vi "ActuatorMotor.vi"(4 "Actuator Name":string, 5 "Command":T1(ring)=enum."GetAbsolutePosition", 6 "error in (no error)":errorcluster, 8 "Y":dbl, 9 "X":dbl) -> (0 "error out":errorcluster, 2 "Y out":dbl, 3 "X out":dbl)   [LabVIEW 2009]
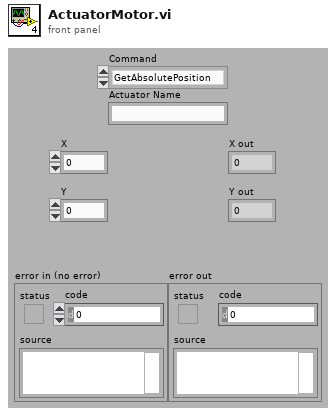
[diagram p1: front panel]
types:
  T1 = enum16{"Acquire", "GetAbsolutePosition", "AbsoluteMove", "Release"}
  T2 = typedef "MotorStatus.ctl" = cluster{"Managed?":bool, "Position":i32, "Name":string, "Status":enum16{"OFF", "IDLE", "MOVING", "HOMING"}}
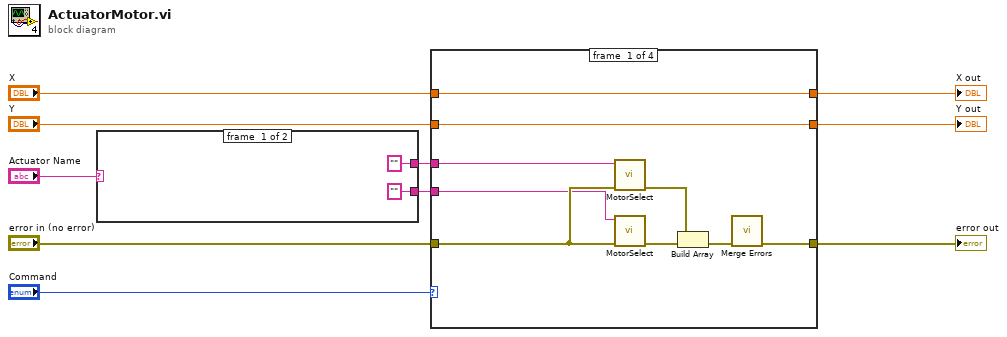
[diagram p0: block diagram]
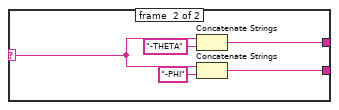
[diagram p2: hidden frame]
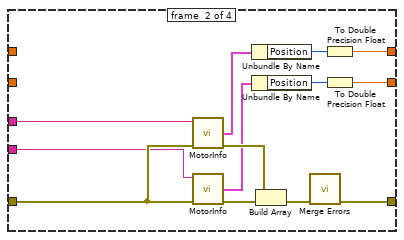
[diagram p3: hidden frame]
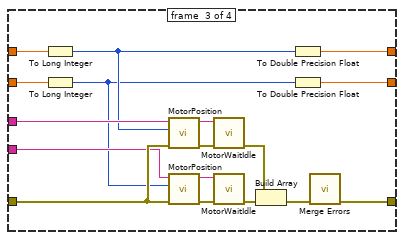
[diagram p4: hidden frame]
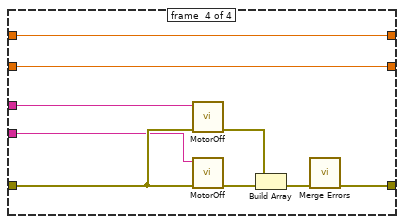
[diagram p5: hidden frame]
diagram:
  n1 = case shown="Default" "Actuator Name" {
    selector: "Actuator Name" -> [_ w15]
    tunnel: ["" w14] -> w4
    tunnel: ["" w13] -> w3
    frame #0 {
    }
    frame #1 {
      n2 = Concatenate Strings(w15, "-THETA" ("string")) -> (w14:string)
      n3 = Concatenate Strings(w15, "-PHI" ("string")) -> (w13:string)
    }
  }
  n4 = case shown="\"AbsoluteMove\"" "Command" {
    tunnel: "error in (no error)" -> [w26 w39 w56 w65]
    tunnel: [w23 w36 w40 w62] -> w9
    tunnel: "X" -> [w19 _ w52 w58]
    tunnel: "Y" -> [w18 _ w51 w57]
    tunnel: w4 -> [w21 w34 w54 w60]
    tunnel: w3 -> [w20 w33 w53 w59]
    tunnel: [w19 w28 w49 w58] -> w2
    tunnel: [w18 w27 w47 w57] -> w1
    frame #0 {
      n5 = call "MotorSelect.vi"("Motor"=w21, "error in (no error)"=w26) -> ("error out"=w24:errorcluster)  [unwired: 6 in, 1 out]
      n6 = call "MotorSelect.vi"("Motor"=w20, "error in (no error)"=w26) -> ("error out"=w25:errorcluster)  [unwired: 6 in, 1 out]
      n7 = Build Array(w24, w25) -> (w22:errorcluster[])
      n8 = call <vilib>:"Merge Errors.vi"("error array in"=w22) -> ("error out"=w23:errorcluster)  [unwired: 6 in]
    }
    frame #1 {
      n9 = call "MotorInfo.vi"("error in (no error)"=w39, "Motor"=w34) -> ("error out"=w37:errorcluster, "Axis status"=w32:T2)  [unwired: 5 in, 1 out]
      n10 = call "MotorInfo.vi"("error in (no error)"=w39, "Motor"=w33) -> ("error out"=w38:errorcluster, "Axis status"=w31:T2)  [unwired: 5 in, 1 out]
      n11 = Unbundle By Name(w32) -> ("Position"=w30:i32)
      n12 = Unbundle By Name(w31) -> ("Position"=w29:i32)
      n13 = Build Array(w37, w38) -> (w35:errorcluster[])
      n14 = call <vilib>:"Merge Errors.vi"("error array in"=w35) -> ("error out"=w36:errorcluster)  [unwired: 6 in]
      n15 = To Double Precision Float(number=w30) -> (double precision float=w28:dbl)
      n16 = To Double Precision Float(number=w29) -> (double precision float=w27:dbl)
    }
    frame #2 {
      n17 = To Long Integer(number=w52) -> (32bit integer=w50:i32)
      n18 = To Long Integer(number=w51) -> (32bit integer=w48:i32)
      n19 = call "MotorPosition.vi"("Motor"=w54, "Position"=w50, "error in (no error)"=w56) -> ("Motor out"=w46:string, "error out"=w45:errorcluster)  [unwired: 5 in]
      n20 = call "MotorPosition.vi"("Motor"=w53, "Position"=w48, "error in (no error)"=w56) -> ("Motor out"=w44:string, "error out"=w43:errorcluster)  [unwired: 5 in]
      n21 = call "MotorWaitIdle.vi"("Motor"=w46, "error in (no error)"=w45) -> ("error out"=w41:errorcluster)  [unwired: 6 in, 1 out]
      n22 = call "MotorWaitIdle.vi"("Motor"=w44, "error in (no error)"=w43) -> ("error out"=w42:errorcluster)  [unwired: 6 in, 1 out]
      n23 = Build Array(w41, w42) -> (w55:errorcluster[])
      n24 = To Double Precision Float(number=w50) -> (double precision float=w49:dbl)
      n25 = To Double Precision Float(number=w48) -> (double precision float=w47:dbl)
      n26 = call <vilib>:"Merge Errors.vi"("error array in"=w55) -> ("error out"=w40:errorcluster)  [unwired: 6 in]
    }
    frame #3 {
      n27 = call "MotorOff.vi"("Motor"=w60, "error in (no error)"=w65) -> ("error out"=w63:errorcluster)  [unwired: 6 in, 1 out]
      n28 = call "MotorOff.vi"("Motor"=w59, "error in (no error)"=w65) -> ("error out"=w64:errorcluster)  [unwired: 6 in, 1 out]
      n29 = Build Array(w63, w64) -> (w61:errorcluster[])
      n30 = call <vilib>:"Merge Errors.vi"("error array in"=w61) -> ("error out"=w62:errorcluster)  [unwired: 6 in]
    }
  }
  "error out" <- w9
  "Y out" <- w1
  "X out" <- w2
